vi "接收校验.vi"(1 "字符串":string) -> (0 "s? t:f":string)   [LabVIEW 2016]
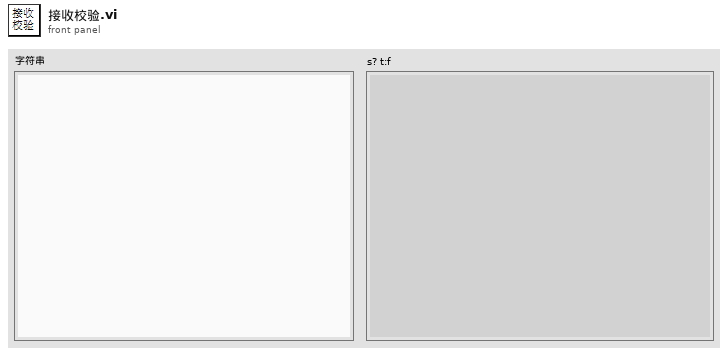
[diagram p1: front panel]
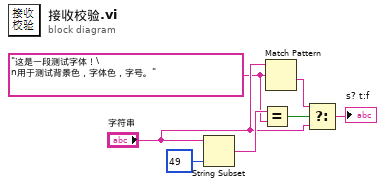
[diagram p0: block diagram]
diagram:
  w1 = "这是一段测试字体！\n用于测试背景色，字体色，字号。" ("接收数据区")
  n1 = String Subset(string="字符串", length (rest)=49 ("长度（剩余）")) -> (substring=w7:string)  [unwired: 1 in]
  n2 = Equal?(x=w7, y=w1) -> (x = y?=w5:bool)
  n3 = Match Pattern(string="字符串", regular expression=w1) -> (after substring=w4:string)  [unwired: 1 in, 3 out]
  n4 = Select(t=w4, s=w5, f="字符串") -> (s? t:f=→"s? t:f":string)
